vi "Switch to WiFi.vi"(7 "Retry wait time [ms]":u32=500, 8 "Error In":errorcluster, 10 "TCP Configuration":T5, 11 "LINX Resource":T1) -> (0 "Error Out":errorcluster, 3 "LINX Resource out":T1)   [LabVIEW 2019, in "LINXx.lvlib"]
doc: "Switch from serial connection to the LINX device to TCP communication. If TCP settings fail, VI continues with original serial connection.\nUse IP address 0.0.0.0 to use DHCP (router assigns address to board)"
uses:
  LINXx.lvlib
  <vilib>/MakerHub/LINX/Private/Device/Type Defs/TCP Config.ctl
  <vilib>/MakerHub/LINX/Private/Type Defs/LINX Ref.ctl
  <vilib>/MakerHub/LINX/Private/Type Defs/Platform.ctl
  <vilib>/MakerHub/LINX/Private/Type Defs/Interface.ctl
  <vilib>/MakerHub/LINX/Private/Device/Type Defs/LINX Device Config.ctl
  <vilib>/MakerHub/LINX/Private/Device/Type Defs/Channels.ctl
  <vilib>/Utility/error.llb/DialogType.ctl
  <vilib>/MakerHub/LINX/Public/Utilities/Open TCP.vi
  <vilib>/MakerHub/LINX/Public/Utilities/Open Serial.vi
  <vilib>/MakerHub/LINX/LMH-LINX.lvlib
  <vilib>/MakerHub/LINX/Private/Device/Device.lvlib
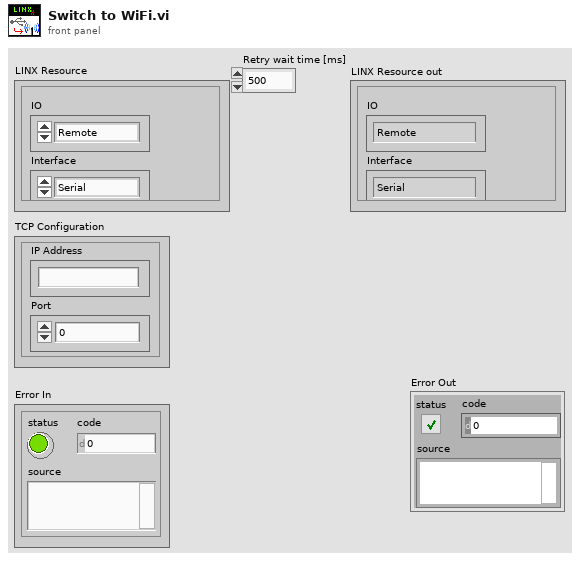
[diagram p1: front panel]
types:
  T1 = typedef "LMH-LINX.lvlib/LINX Ref.ctl" = cluster{"IO":T2, "Interface":T3, "LINX Device Config":T4}
  T2 = typedef "LMH-LINX.lvlib/Platform.ctl" = enum16{"Remote", "Local"}
  T3 = typedef "LMH-LINX.lvlib/Interface.ctl" = enum16{"Serial", "TCP"}
  T4 = typedef "LMH-LINX.lvlib/Device.lvlib/LINX Device Config.ctl" = cluster{"Interface":T3, "COM Port":refnum<visa-resource-name>, "TCP Configuration":T5, "Device Family":u8, "Device ID":u8, "Device Name":string, "TCP Ref":refnum<k5>, "Channels":T6}
  T5 = typedef "LMH-LINX.lvlib/Device.lvlib/TCP Config.ctl" = cluster{"IP Address":string, "Port":u16}
  T6 = typedef "LMH-LINX.lvlib/Channels.ctl" = cluster{"DI":u8[], "DO":u8[], "AI":u8[], "AO":u8[], "PWM":u8[], "QE":u8[], "UART":u8[], "I2C 2":u8[], "SPI":u8[], "CAN":u8[], "Servo":u8[], "AI Ref (V)":dbl, "AI Resolution (Bits)":u8, "AO Ref (V)":dbl, "AO Resolution (Bits)":u8}
  T7 = typedef "DialogType.ctl" = u16
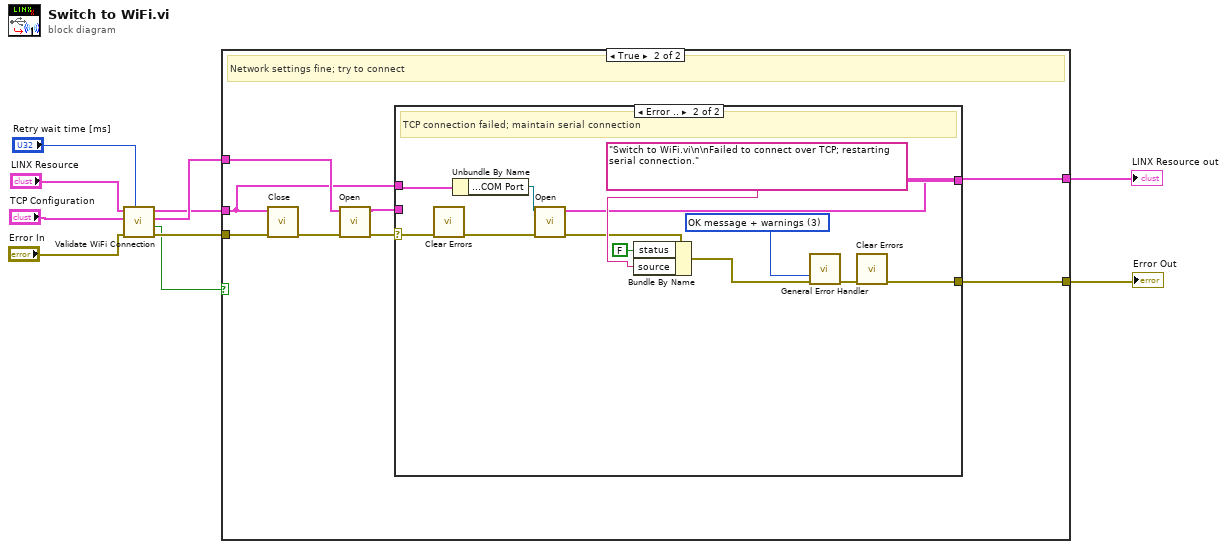
[diagram p0: block diagram]
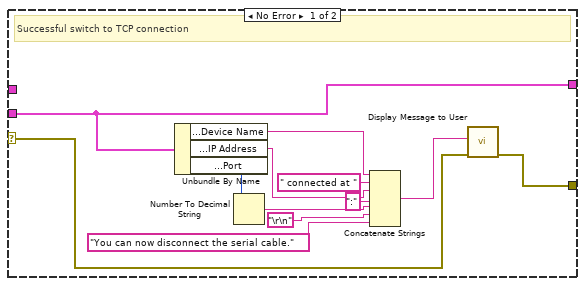
[diagram p3: hidden frame]
diagram:
  n1 = call "Validate WiFi Connection.vi"("Retry wait time [ms]"="Retry wait time [ms]", "Error In"="Error In", "TCP Configuration"="TCP Configuration", "LINX Resource"="LINX Resource") -> ("error out"=w8:errorcluster, "Connected?"=w1:bool, "TCP Config out"=w7:T5, "LINX Resource Out"=w3:T1)  [unwired: 4 in]
  n2 = case shown="True" w1 {
    tunnel: [w12 w18] -> w10
    tunnel: [w11 w17] -> w9
    tunnel: w8 -> [w11 w14]
    tunnel: w7 -> [_ w16]
    tunnel: w3 -> [w12 w15]
    frame False {
      # "No connection to network; continue on"
    }
    frame True {
      # "Network settings fine; try to connect"
      n3 = call <vilib>:"Close.vi"("Error In"=w14, "LINX Resource"=w15) -> ("Error Out"=w13:errorcluster)  [unwired: 9 in]
      n4 = call-poly <vilib>:"Open.vi"("Error In"=w13, "TCP Configuration"=w16) -> ("Error Out"=w20:errorcluster, "LINX Resource"=w19:T1)  [unwired: 7 in, 1 out]
      n5 = case shown="Error .." w20 {
        selector: w20 -> [w21 w34]
        tunnel: [w32 w38] -> w18
        tunnel: w19 -> [w32 _]
        tunnel: [w23 w39] -> w17
        tunnel: w15 -> [_ w37]
        frame No Error {
          # "Successful switch to TCP connection"
          n6 = Unbundle By Name(w32) -> ("LINX Device Config.Device Name"=w31:string, "LINX Device Config.TCP Configuration.IP Address"=w29:string, "LINX Device Config.TCP Configuration.Port"=w27:u16)
          n7 = Number To Decimal String(number=w27) -> (decimal integer string=w26:string)  [unwired: 1 in]
          n8 = Concatenate Strings(w31, " connected at " ("string"), w29, ":" ("string"), w26, "\r\n", "You can now disconnect the serial cable." ("string")) -> (w22:string)
          n9 = call "Display Message to User"("error in (no error)"=w21, "Message"=w22) -> ("error out"=w23:errorcluster)  [unwired: 8 in, 1 out]
        }
        frame Error {
          w42 = T7 3 items=["no dialog", "OK message", "continue or stop message", "OK message + warnings", "continue/stop + warnings"] ("type of dialog (OK msg:1)")
          # "TCP connection failed; maintain serial connection"
          n10 = call <vilib>:"Clear Errors.vi"("error in (no error)"=w34) -> ("error out"=w33:errorcluster)  [unwired: 5 in, 1 out]
          n11 = Unbundle By Name(w37) -> ("LINX Device Config.COM Port"=w36:refnum<visa-resource-name>)
          n12 = call-poly <vilib>:"Open.vi"("Error In"=w33, "Serial Port"=w36) -> ("Error Out"=w35:errorcluster, "LINX Resource"=w38:T1)  [unwired: 7 in, 1 out]
          n13 = Bundle By Name(cluster=w35, "status"=FALSE, "source"="Switch to WiFi.vi\n\nFailed to connect over TCP; restarting serial connection." ("string")) -> (w41:errorcluster)
          n14 = call <vilib>:"General Error Handler.vi"("type of dialog (OK msg:1)"=w42, "error in (no error)"=w41) -> ("error out"=w40:errorcluster)  [unwired: 9 in, 4 out]
          n15 = call <vilib>:"Clear Errors.vi"("error in (no error)"=w40) -> ("error out"=w39:errorcluster)  [unwired: 5 in, 1 out]
        }
      }
    }
  }
  "Error Out" <- w9
  "LINX Resource out" <- w10
